vi "Actor Core.vi"(8 "error in":errorcluster, 11 "ConcreteModel in":refnum<class "ConcreteModel.lvclass">) -> (0 "error out":errorcluster, 3 "Actor out":refnum<class "Actor.lvclass">)   [LabVIEW 2015, in "TopLevelApplication.lvlib" / "ConcreteModel.lvclass"]
doc: "(<B>Filename</B>: Actor Framework.lvlib:Actor.lvclass:Actor Core.vi)\n\nReceives messages to the actor, reacts to them, and initiates any error handling that may shut the actor down.\n\nDescendant classes may override this VI to append parallel tasks for the actor to complete while it handles messages. Overrides use the Call Parent Method node.\n\n<License>\nCopyright © 2017 Composed Systems, LLC | All rights reserved\nwww.composed.io\n\nAuthor: Ethan Stern <ethan.stern@composed.io>\n\nThis software is provided \"AS IS\" WITHOUT WARRANTIES, either express or implied, AND IS FOR EDUCATIONAL PURPOSES ONLY.\n</License>"
uses:
  ConcreteModel.lvclass
  <vilib>/ActorFramework/Actor/Actor.lvclass
  Framework/Mediator/MediatorBusMonitor/MediatorBusMonitor.lvclass
  Framework/IViewable/IViewable/View Position Enum.ctl
  Framework/IViewable/IViewable Messages/Open View Msg/Open View Msg.lvclass/Open View Msg.ctl
  <vilib>/ActorFramework/Message Enqueuer/Message Enqueuer.lvclass/Message Enqueuer.ctl
  Framework/IModel/IModel/IModel.lvclass/IModel.ctl
  Framework/AbstractMessages/PreAddressedMsg/PreAddressedMsg.lvclass/PreAddressedMsg.ctl
  Framework/IMediator/IMediator Messages/Publish Msg/Publish Msg.lvclass/Publish Msg.ctl
  <vilib>/ActorFramework/Message Enqueuer/Enqueue.vi
  Framework/IMediator/IMediator Messages/Publish Msg/Send Pre-Addressed Publish.vi
  Framework/AbstractMessages/PreAddressedMsg/Read Return Address.vi
  <vilib>/ActorFramework/Message Priority Queue/Priority Enqueue.vi
  Framework/IViewable/IViewable Messages/Open View Msg/Open View Msg.lvclass
  Framework/IModel/IModel/IModel.lvclass
  Framework/IViewable/IViewable/IViewable.lvclass
panel:
  in  "User Value (Testing)":dbl=100.0 format="%#_13g"
  in  "Publish Period [ms]":u32=100
  in  "Stop Button":bool
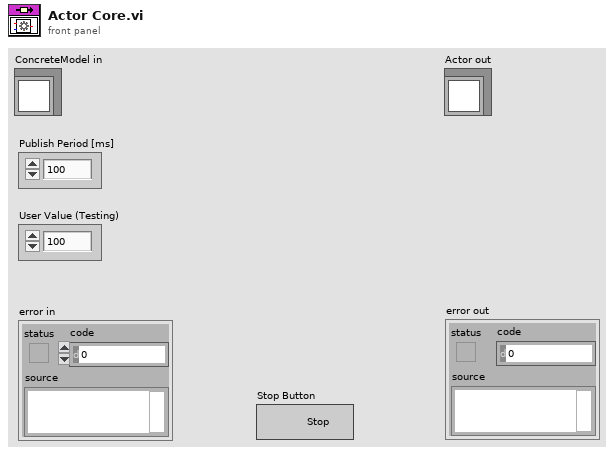
[diagram p1: front panel]
types:
  T1 = typedef "IViewable.lvlib/IViewable.lvclass/View Position Enum.ctl" = enum16{"Centered", "Maximized", "Minimized", "Custom", "Unchanged"}
  T2 = cluster{"seconds since 1Jan1904":timestamp, "number: 0 to 1":dbl}
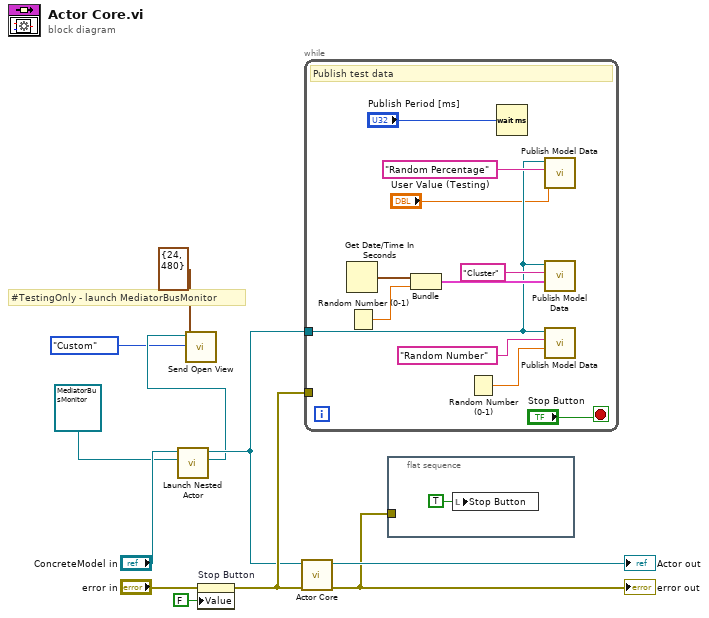
[diagram p0: block diagram]
diagram:
  # "#TestingOnly - launch MediatorBusMonitor"
  n1 = call <vilib>:"Launch Nested Actor.vi"("Nested Actor"=refnum<class "MediatorBusMonitor.lvclass"> refnum ("Mediator.lvlib:MediatorBusMonitor.lvclass"), "Caller Actor in"="ConcreteModel in") -> ("Nested Actor's Enqueuer"=w3:refnum<class "Message Enqueuer.lvclass">, "Caller Actor out"=w6:refnum<class "ConcreteModel.lvclass">)  [unwired: 7 in, 1 out]
  n2 = call "Send Open View.vi"("Custom Position"=cluster{"Top":i16, "Left":i16} {"Top"=24, "Left"=480}, "Position"=View_Position_Enum."Custom", "Message Enqueuer"=w3) -> ()  [unwired: 7 in, 2 out]
  n3 = property on="Stop Button" class="Bool (strict)"(error in="error in", "Value"=FALSE ("Stop Button")) -> (error out=w8:errorcluster)  [unwired: 1 in, 1 out]
  n4 = call-parent "Actor Core.vi"("error in"=w8, "Actor in"=w6) -> ("error out"=w7:errorcluster, "Actor out"=→"Actor out":refnum<class "Actor.lvclass">)  [unwired: 8 in]
  "error out" <- w7
  n5 = while {
    tunnel: w8 -> [_]
    tunnel: w6 -> [w13]
    stop <- "Stop Button" stop-if-true
    # "Publish test data"
    n6 = Get Date/Time In Seconds() -> (seconds since 1Jan1904=w17:timestamp)
    n7 = Random Number (0-1)() -> (number: 0 to 1=w18:dbl)
    n8 = Bundle("seconds since 1Jan1904"=w17, "number: 0 to 1"=w18) -> (w16:T2)  [unwired: 1 in]
    n9 = Random Number (0-1)() -> (number: 0 to 1=w20:dbl)
    n10 = Wait (ms)(milliseconds to wait="Publish Period [ms]") -> ()  [unwired: 1 out]
    n11 = call "Publish Model Data.vi"("Data to Publish"="User Value (Testing)", "Topic Name"="Random Percentage", "IModel in"=w13) -> ()  [unwired: 7 in, 2 out]
    n12 = call "Publish Model Data.vi"("Data to Publish"=w16, "Topic Name"="Cluster", "IModel in"=w13) -> ()  [unwired: 7 in, 2 out]
    n13 = call "Publish Model Data.vi"("Data to Publish"=w20, "Topic Name"="Random Number", "IModel in"=w13) -> ()  [unwired: 7 in, 2 out]
  }
  n14 = flat-sequence {
    tunnel: w7 -> [_]
    frame #0 {
      n15 = local write "Stop Button"(TRUE ("Stop Button")) -> ()
    }
  }
